vi "Parse Variant.vi"(8 "error in":errorcluster, 10 "variant":variant) -> (0 "error out":errorcluster, 1 "Types":T1[](array[typedef]), 2 "Strings":string[](array[string]), 3 "Variants":variant[](array[variant]), 4 "Types (strings)":string[](array[string]))   [LabVIEW 2016, in "LV-Data.PGSQL.lvclass"]
uses:
  LV-Data.PGSQL.lvclass
  <vilib>/Utility/Data Type/Type Definitions/Data Type.ctl
  Typedefs/Errors--enum.ctl
  <vilib>/Utility/Data Type/NI_Data Type.lvlib
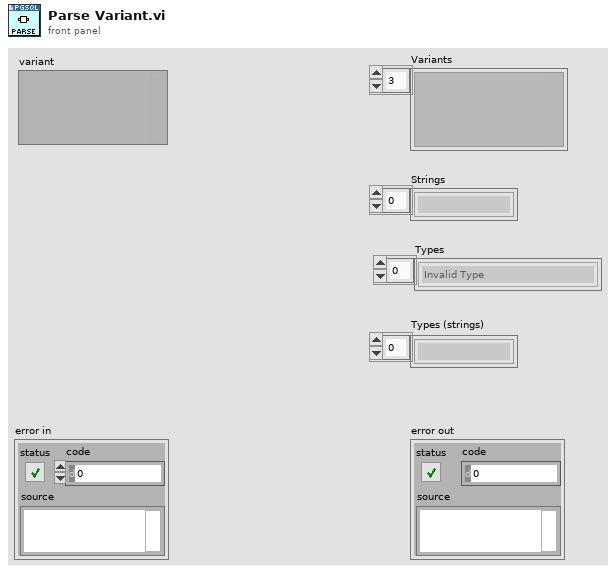
[diagram p1: front panel]
types:
  T1 = typedef "NI_Data Type.lvlib/Data Type.ctl" = enum8{"Invalid Type", "Void", "I8", "I16", "I32", "I64", "U8", "U16", "U32", "U64", "Single Float", "Double Float", "Extended Float", "Single Complex", "Double Complex", "Extended Complex", "Enum U8", "Enum U16", "Enum U32", "Enum U64", "Single Float With Unit", "Double Float With Unit", "Extended Float With Unit", "Single Complex with Unit", "Double Complex with Unit", "Extended Complex with Unit", "Boolean", "String", "Path", "Picture", "Tag", "Array", "Cluster", "Variant", "LV Variant", "Waveform", "Timestamp", "Digital Waveform", "Digital Data", "ExpressData", "Refnum", "External Data", "VI", "Poly VI", "LabVIEW Class Instance", "Fixed Point"}
  T2 = typedef "LV-Data.PGSQL.lvclass/Errors--enum.ctl" = enum16{"0: None", "5005: Path Type Not Supported", "5006: Number of Variables", "5008: Cannot write two data points", "5030: Start and End Times Identical", "5031: Input is not wholly", "5033: Bad path or paths", "5040: Invalid Instrument Name", "5050: Column can only hold string", "5051 Column can only hold bool", "5052: Column can only hold double", "5053: Column can only hold int"}
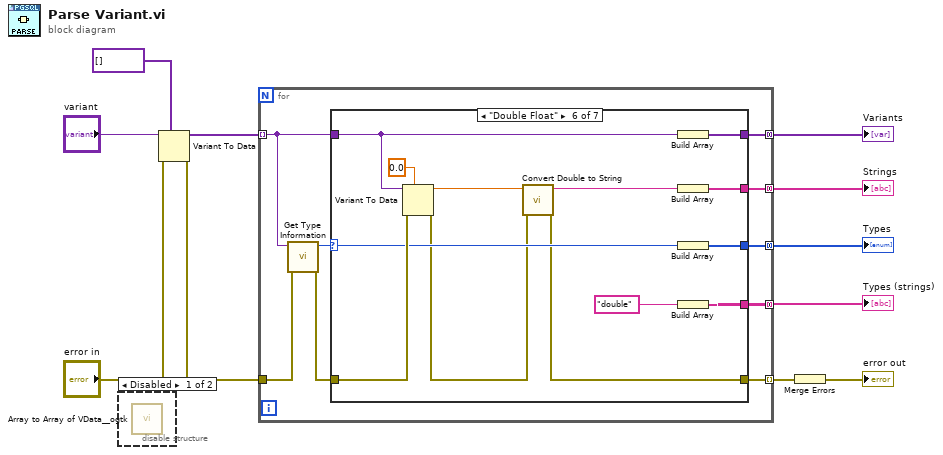
[diagram p0: block diagram]
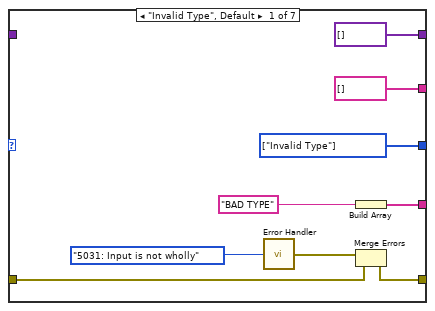
[diagram p3: hidden frame]
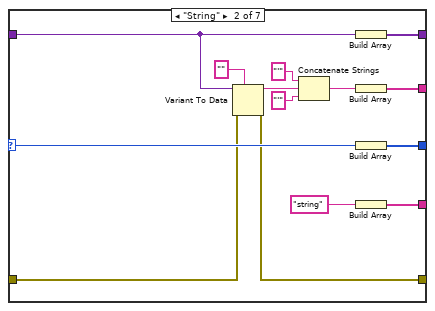
[diagram p4: hidden frame]
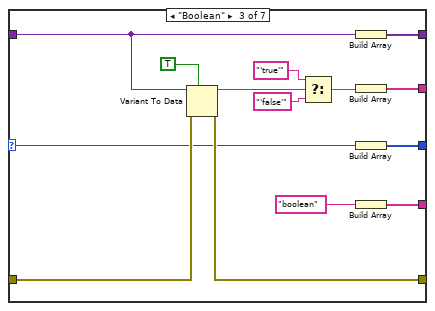
[diagram p5: hidden frame]
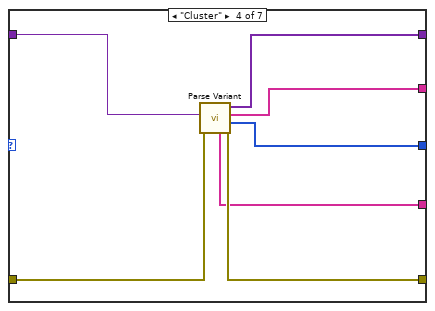
[diagram p6: hidden frame]
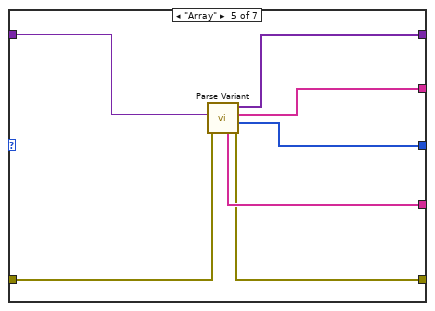
[diagram p7: hidden frame]
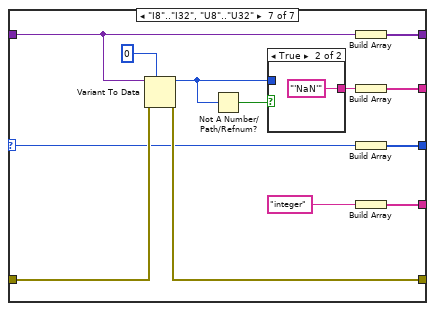
[diagram p8: hidden frame]
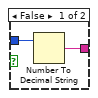
[diagram p9: hidden frame]
diagram:
  n1 = disable-structure shown="Disabled" {
    frame Disabled {
      n2 = call <userlib>:"Array to Array of VData__ogtk.vi"() -> ()  [unwired: 10 in, 2 out]
    }
    frame Enabled {
    }
  }
  n3 = Variant To Data(error in="error in", type=variant[] [], Variant="variant") -> (data=w2:variant[], error out=w1:errorcluster)
  n4 = for {
    tunnel: w2 -> [w15] mode=indexing
    tunnel: [w19] -> w11 mode=concatenating
    tunnel: [w18] -> w10 mode=concatenating
    tunnel: [w17] -> w9 mode=concatenating
    tunnel: [w12] -> w7 mode=indexing
    tunnel: w1 -> [w14]
    tunnel: [w16] -> w6 mode=concatenating
    n5 = call <vilib>:"Get Type Information.vi"("error in (no error)"=w14, "Variant"=w15) -> ("error out"=w13:errorcluster, "Type"=w20:T1)  [unwired: 5 in, 3 out]
    n6 = case shown="\"Double Float\"" w20 {
      selector: w20 -> [_ w32 w44 _ _ w75 w88]
      tunnel: w15 -> [_ w36 w50 w64 w71 w79 w85]
      tunnel: [string[] [] ("Strings") w38 w52 w59 w70 w82 w94] -> w18
      tunnel: [w27 w37 w51 w60 w65 w83 w96] -> w19
      tunnel: [variant[] [] ("Variants") w35 w49 w58 w66 w80 w95] -> w17
      tunnel: [w26 w33 w47 w61 w69 w77 w91] -> w16
      tunnel: w13 -> [w24 w31 w46 w63 w68 w76 w90]
      tunnel: [w23 w30 w45 w62 w67 w72 w89] -> w12
      frame "Invalid Type", Default {
        w27 = T1[] [enum."Invalid Type"] items=["Invalid Type", "Void", "I8", "I16", "I32", "I64", "U8", "U16", "U32", "U64", "Single Float", "Double Float", "Extended Float", "Single Complex", "Double Complex", "Extended Complex", "Enum U8", "Enum U16", "Enum U32", "Enum U64", "Single Float With Unit", "Double Float With Unit", "Extended Float With Unit", "Single Complex with Unit", "Double Complex with Unit", "Extended Complex with Unit", "Boolean", "String", "Path", "Picture", "Tag", "Array", "Cluster", "Variant", "LV Variant", "Waveform", "Timestamp", "Digital Waveform", "Digital Data", "ExpressData", "Refnum", "External Data", "VI", "Poly VI", "LabVIEW Class Instance", "Fixed Point"] ("Types")
        n7 = call "Error Handler.vi"("Error code"=Errors--enum."5031: Input is not wholly") -> ("error out"=w21:errorcluster)
        n8 = Build Array("BAD TYPE") -> (w26:string[])
        n9 = Merge Errors(w21, w24) -> (w23:errorcluster)
      }
      frame "String" {
        n10 = Variant To Data(error in=w31, type="", Variant=w36) -> (data=w42:string, error out=w30:errorcluster)
        n11 = Concatenate Strings("'" ("string"), w42, "'" ("string")) -> (w39:string)
        n12 = Build Array(w36) -> (w35:variant[])
        n13 = Build Array(w39) -> (w38:string[])
        n14 = Build Array(w32) -> (w37:T1[])
        n15 = Build Array("string") -> (w33:string[])
      }
      frame "Boolean" {
        n16 = Variant To Data(error in=w46, type=TRUE, Variant=w50) -> (data=w56:bool, error out=w45:errorcluster)
        n17 = Select(t="'true'", s=w56, f="'false'") -> (s? t:f=w53:string)
        n18 = Build Array(w50) -> (w49:variant[])
        n19 = Build Array(w53) -> (w52:string[])
        n20 = Build Array(w44) -> (w51:T1[])
        n21 = Build Array("boolean") -> (w47:string[])
      }
      frame "Cluster" {
        n22 = call "Parse Variant.vi"("error in"=w63, "variant"=w64) -> ("error out"=w62:errorcluster, "Types"=w60:T1[], "Strings"=w59:string[], "Variants"=w58:variant[], "Types (strings)"=w61:string[])  [unwired: 5 in]
      }
      frame "Array" {
        n23 = call "Parse Variant.vi"("error in"=w68, "variant"=w71) -> ("error out"=w67:errorcluster, "Types"=w65:T1[], "Strings"=w70:string[], "Variants"=w66:variant[], "Types (strings)"=w69:string[])  [unwired: 5 in]
      }
      frame "Double Float" {
        n24 = Variant To Data(error in=w76, type=0.0, Variant=w79) -> (data=w74:dbl, error out=w73:errorcluster)
        n25 = call "Convert Double to String.vi"("error in"=w73, "Numeric"=w74) -> ("error out"=w72:errorcluster, "PGSQL String"=w81:string)  [unwired: 8 in]
        n26 = Build Array(w79) -> (w80:variant[])
        n27 = Build Array(w81) -> (w82:string[])
        n28 = Build Array(w75) -> (w83:T1[])
        n29 = Build Array("double") -> (w77:string[])
      }
      frame "I8".."I32", "U8".."U32" {
        n30 = Variant To Data(error in=w90, type=0, Variant=w85) -> (data=w86:i32, error out=w89:errorcluster)
        n31 = Not A Number/Path/Refnum?(number/path/refnum=w86) -> (NaN/Path/Refnum?=w87:bool)
        n32 = case shown="True" w87 {
          tunnel: [w99 "'NaN'"] -> w93
          tunnel: w86 -> [w98 _]
          frame False {
            n33 = Number To Decimal String(number=w98) -> (decimal integer string=w99:string)  [unwired: 1 in]
          }
          frame True {
          }
        }
        n34 = Build Array(w85) -> (w95:variant[])
        n35 = Build Array(w93) -> (w94:string[])
        n36 = Build Array(w88) -> (w96:T1[])
        n37 = Build Array("integer") -> (w91:string[])
      }
    }
  }
  "Variants" <- w9
  "Types" <- w11
  "Strings" <- w10
  "Types (strings)" <- w6
  n38 = Merge Errors(w7) -> (→"error out":errorcluster)
